vi "主介面.vi"() -> ()   [LabVIEW 2022 SP3]
panel:
  in  "最高權限":bool
  in  "關閉":bool
  in  "登入":bool
  in  "輸入使用者密碼:":string
  in  "輸入使用者帳號:":string
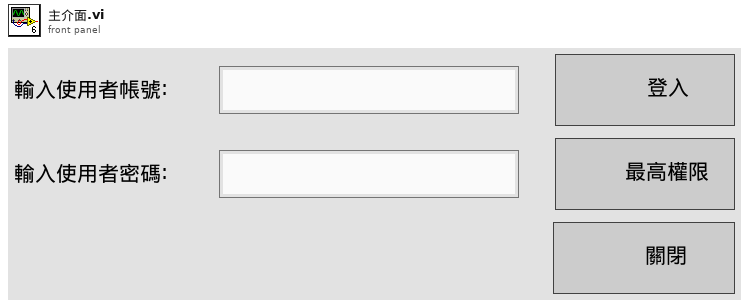
[diagram p1: front panel]
types:
  T1 = typedef "主介面Control.ctl" = enum16{"進入主程式", "初始", "登入", "最高權限模式", "關閉"}
  T2 = enum16{"open", "replace", "create", "open or create", "replace or create", "replace or create with confirmation"}
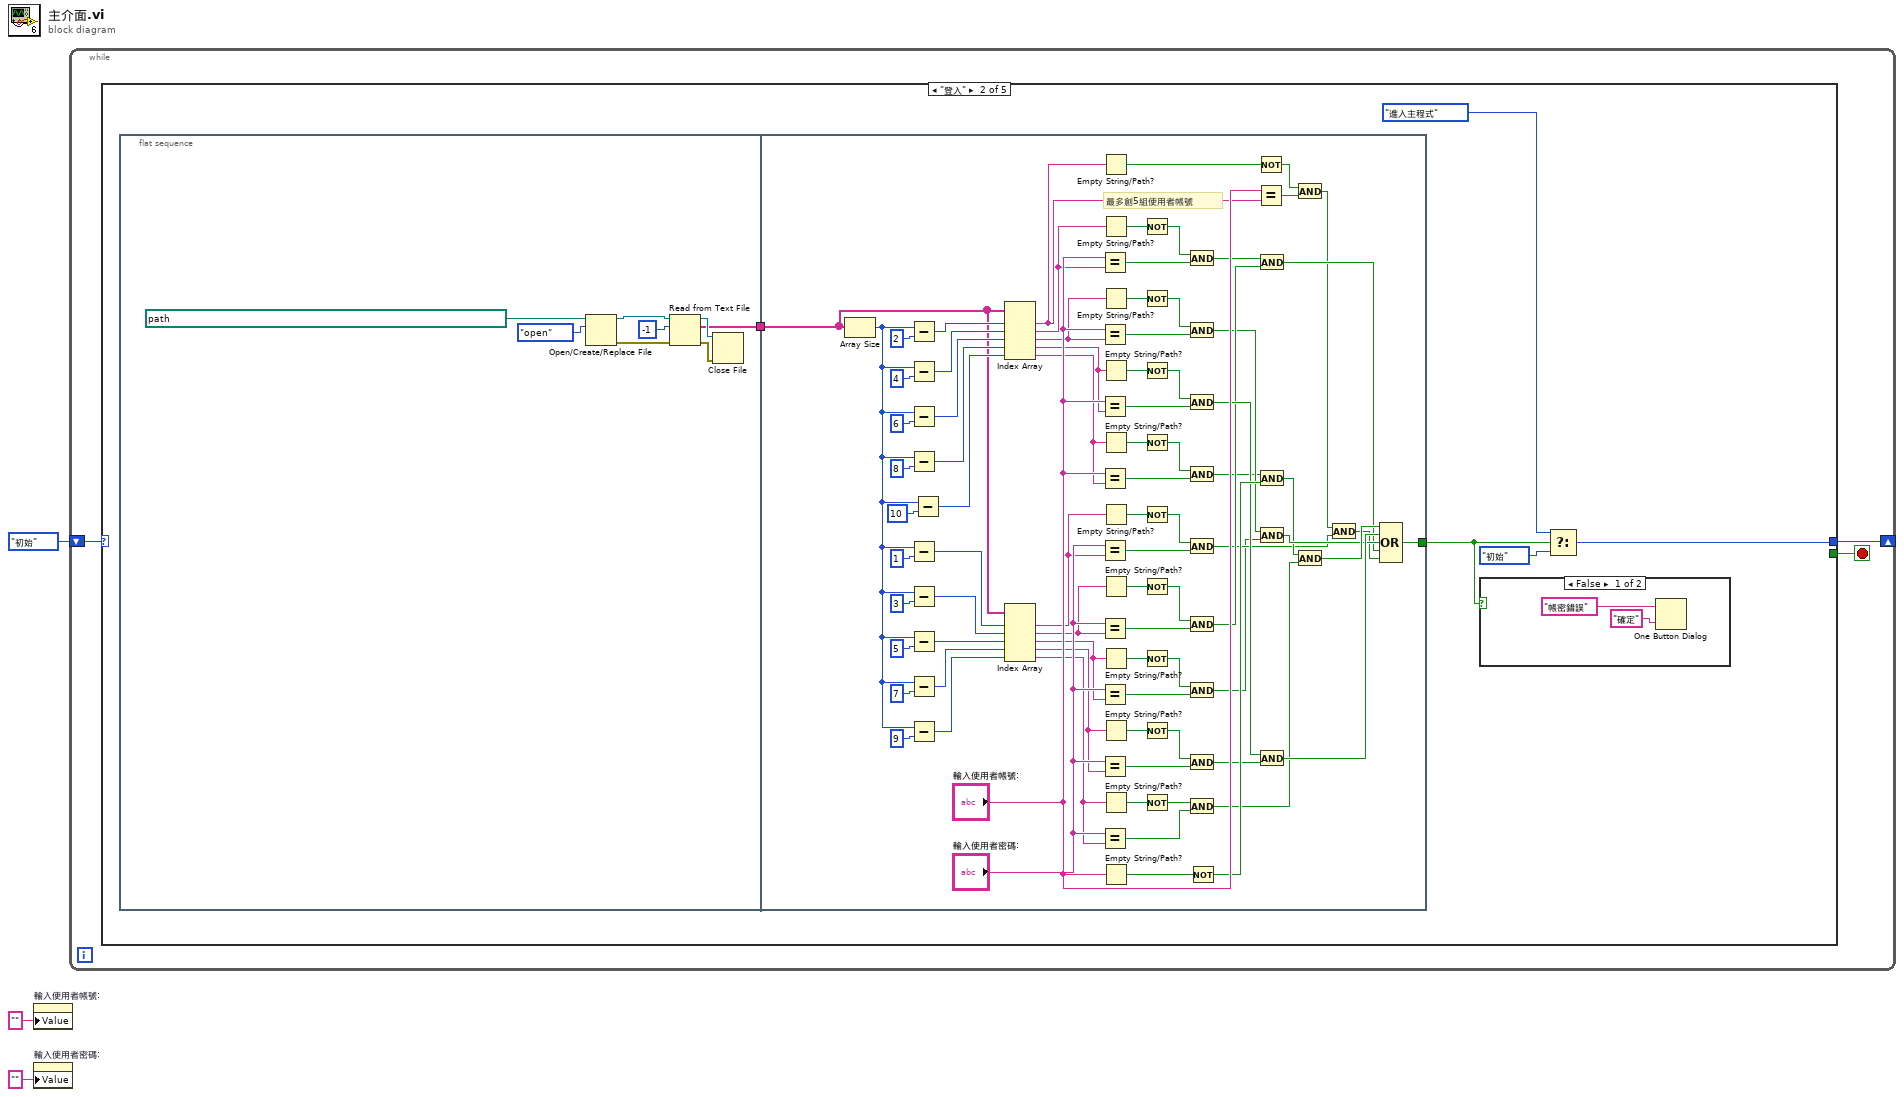
[diagram p0: block diagram]
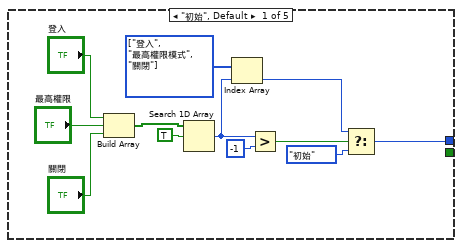
[diagram p2: hidden frame]
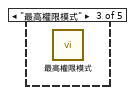
[diagram p4: hidden frame]
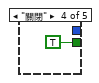
[diagram p5: hidden frame]
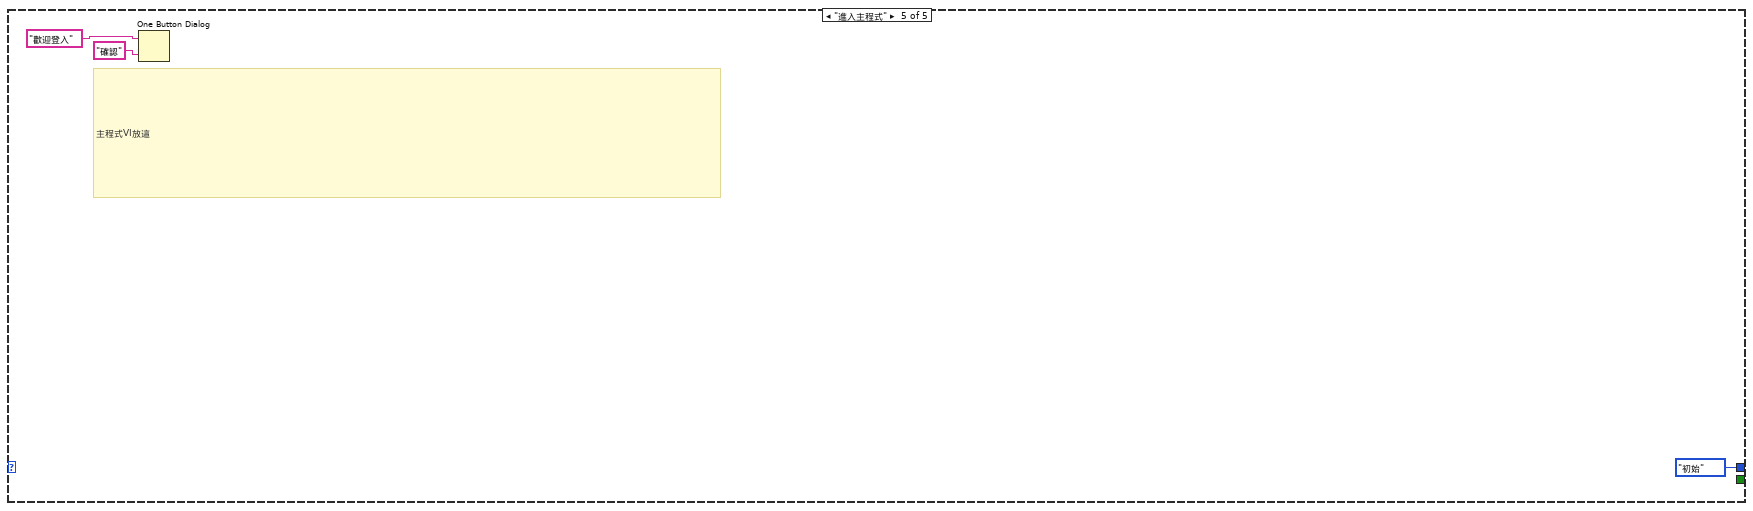
[diagram p6: hidden frame]
diagram:
  n1 = property on="輸入使用者帳號:" class="Str"("Value"="" ("輸入使用者帳號:")) -> ()  [unwired: 2 in, 2 out]
  n2 = property on="輸入使用者密碼:" class="Str"("Value"="" ("輸入使用者密碼:")) -> ()  [unwired: 2 in, 2 out]
  n3 = while {
    shift-right: [w5] -> _
    shift-left: 主介面Control."初始" -> [w6]
    stop <- w4 stop-if-true
    n4 = case shown="\"登入\"" w6 {
      tunnel: [w7 w21 _ _ 主介面Control."初始"] -> w5
      tunnel: [_ _ _ TRUE _] -> w4
      frame "初始", Default {
        w13 = T1[] [enum."登入", enum."最高權限模式", enum."關閉"] items=["進入主程式", "初始", "登入", "最高權限模式", "關閉"]
        n5 = Build Array("登入", "最高權限", "關閉") -> (w15:bool[])
        n6 = Search 1D Array(1D array=w15, element=TRUE) -> (index of element=w12:i32)  [unwired: 1 in]
        n7 = Index Array(array=w13, index=w12) -> (element=w9:T1)
        n8 = Greater?(x=w12, y=-1) -> (0:w10:bool)
        n9 = Select(t=w9, s=w10, f=主介面Control."初始") -> (s? t:f=w7:T1)
      }
      frame "登入" {
        n10 = flat-sequence {
          tunnel: [w27] -> w23
          tunnel: w23 -> [w106]
          tunnel: [w88] -> w19
          frame #0 {
            n11 = Open/Create/Replace File(file path (use dialog)=path "D:/Project/Semiconductor Equipment/機械手臂/使用者帳密.txt", operation (0:open)=T2."open") -> (refnum out=w33:refnum<file>, error out=w30:errorcluster)  [unwired: 4 in, 1 out]
            n12 = Read from Text File(file (use dialog)=w33, count=-1, error in=w30) -> (refnum out=w32:refnum<file>, text=w27:string[], error out=w31:errorcluster)  [unwired: 1 in, 1 out]
            n13 = Close File(refnum=w32, error in=w31) -> ()  [unwired: 2 out]
          }
          frame #1 {
            # "最多創5組使用者帳號"
            n14 = Array Size(array=w106) -> (size(s)=w105:i32)
            n15 = Subtract(x=w105, y=2) -> (x-y=w111:i32)
            n16 = Subtract(x=w105, y=4) -> (x-y=w110:i32)
            n17 = Subtract(x=w105, y=6) -> (x-y=w109:i32)
            n18 = Subtract(x=w105, y=8) -> (x-y=w108:i32)
            n19 = Subtract(x=w105, y=1) -> (x-y=w99:i32)
            n20 = Subtract(x=w105, y=3) -> (x-y=w98:i32)
            n21 = Subtract(x=w105, y=5) -> (x-y=w97:i32)
            n22 = Subtract(x=w105, y=7) -> (x-y=w96:i32)
            n23 = Subtract(x=w105, y=9) -> (x-y=w95:i32)
            n24 = Subtract(x=w105, y=10) -> (x-y=w107:i32)
            n25 = Index Array(array=w106, index #1=w111, index #2=w110, index #3=w109, index #4=w108, index #5=w107) -> (element #1=w52:string, element #2=w58:string, element #3=w43:string, element #4=w78:string, element #5=w37:string)
            n26 = Index Array(array=w106, index #1=w99, index #2=w98, index #3=w97, index #4=w96, index #5=w95) -> (element #1=w49:string, element #2=w55:string, element #3=w44:string, element #4=w69:string, element #5=w79:string)
            n27 = Equal?(x="輸入使用者帳號:", y=w58) -> (x = y?=w57:bool)
            n28 = Equal?(x="輸入使用者帳號:", y=w43) -> (x = y?=w42:bool)
            n29 = Equal?(x="輸入使用者帳號:", y=w78) -> (x = y?=w73:bool)
            n30 = Equal?(x="輸入使用者帳號:", y=w37) -> (x = y?=w36:bool)
            n31 = Equal?(x="輸入使用者密碼:", y=w49) -> (x = y?=w48:bool)
            n32 = Equal?(x="輸入使用者密碼:", y=w55) -> (x = y?=w54:bool)
            n33 = Equal?(x="輸入使用者密碼:", y=w44) -> (x = y?=w46:bool)
            n34 = Equal?(x="輸入使用者密碼:", y=w69) -> (x = y?=w68:bool)
            n35 = Equal?(x="輸入使用者密碼:", y=w79) -> (x = y?=w81:bool)
            n36 = Empty String/Path?(string/path=w52) -> (empty?=w64:bool)
            n37 = Empty String/Path?(string/path=w58) -> (empty?=w71:bool)
            n38 = Empty String/Path?(string/path=w43) -> (empty?=w40:bool)
            n39 = Empty String/Path?(string/path=w78) -> (empty?=w77:bool)
            n40 = Empty String/Path?(string/path=w37) -> (empty?=w39:bool)
            n41 = Empty String/Path?(string/path=w49) -> (empty?=w61:bool)
            n42 = Empty String/Path?(string/path=w55) -> (empty?=w65:bool)
            n43 = Empty String/Path?(string/path=w44) -> (empty?=w34:bool)
            n44 = Empty String/Path?(string/path=w69) -> (empty?=w74:bool)
            n45 = Empty String/Path?(string/path=w79) -> (empty?=w83:bool)
            n46 = Empty String/Path?(string/path="輸入使用者帳號:") -> (empty?=w86:bool)
            n47 = Not(x=w71) -> (.not. x?=w70:bool)
            n48 = Not(x=w40) -> (.not. x?=w59:bool)
            n49 = Not(x=w77) -> (.not. x?=w76:bool)
            n50 = Not(x=w39) -> (.not. x?=w38:bool)
            n51 = Not(x=w61) -> (.not. x?=w62:bool)
            n52 = Not(x=w65) -> (.not. x?=w66:bool)
            n53 = Not(x=w34) -> (.not. x?=w60:bool)
            n54 = Not(x=w74) -> (.not. x?=w75:bool)
            n55 = Not(x=w83) -> (.not. x?=w82:bool)
            n56 = And(x=w70, y=w57) -> (x .and. y?=w56:bool)
            n57 = And(x=w59, y=w42) -> (x .and. y?=w41:bool)
            n58 = And(x=w76, y=w73) -> (x .and. y?=w72:bool)
            n59 = And(x=w38, y=w36) -> (x .and. y?=w35:bool)
            n60 = And(x=w62, y=w48) -> (x .and. y?=w47:bool)
            n61 = And(x=w66, y=w54) -> (x .and. y?=w53:bool)
            n62 = And(x=w60, y=w46) -> (x .and. y?=w45:bool)
            n63 = And(x=w75, y=w68) -> (x .and. y?=w67:bool)
            n64 = And(x=w82, y=w81) -> (x .and. y?=w80:bool)
            n65 = Not(x=w86) -> (.not. x?=w85:bool)
            n66 = Not(x=w64) -> (.not. x?=w63:bool)
            n67 = Equal?(x="輸入使用者帳號:", y=w52) -> (x = y?=w51:bool)
            n68 = And(x=w56, y=w53) -> (x .and. y?=w90:bool)
            n69 = And(x=w35, y=w85) -> (x .and. y?=w84:bool)
            n70 = And(x=w41, y=w45) -> (x .and. y?=w91:bool)
            n71 = And(x=w72, y=w67) -> (x .and. y?=w92:bool)
            n72 = And(x=w63, y=w51) -> (x .and. y?=w50:bool)
            n73 = And(x=w84, y=w80) -> (x .and. y?=w93:bool)
            n74 = And(x=w50, y=w47) -> (x .and. y?=w89:bool)
            n75 = Compound Arithmetic op=OR(w93, w92, w91, w90, w89) -> (w88:bool)
          }
        }
        n76 = case shown="False" w19 {
          frame False {
            n77 = One Button Dialog(message="帳密錯誤", button name ("OK")="確定") -> ()  [unwired: 1 out]
          }
          frame True {
          }
        }
        n78 = Select(t=主介面Control."進入主程式", s=w19, f=主介面Control."初始") -> (s? t:f=w21:T1)
      }
      frame "最高權限模式" {
        n79 = call "最高權限模式.vi"() -> ()  [unwired: 1 in]
      }
      frame "關閉" {
      }
      frame "進入主程式" {
        # "主程式VI放這"
        n80 = One Button Dialog(message="歡迎登入", button name ("OK")="確認") -> ()  [unwired: 1 out]
      }
    }
  }
